vi "From_trubine.vi"(8 "error in (no error)":errorcluster) -> (0 "error out":errorcluster)   [LabVIEW 2022 SP3, in "SI657.lvclass"]
uses:
  SI657.lvclass
  SI656/SI656.lvclass
  SI657.lvclass/SI657.ctl
panel:
  out "Switch Ps-Ps_d":dbl
  out "PG target SP":dbl
  out "PG eff SP":dbl
  out "SI656 out":refnum<class "SI656.lvclass">
  in  "SI656.lvclass":refnum<class "SI656.lvclass">
  in  "Set Params 4":T1
  in  "Set Params 3":T1
  in  "Set Params 2":T1
  in  "Set Params":T1
  out "SI657.lvclass out":refnum<class "SI657.lvclass">
  in  "SI657.lvclass":refnum<class "SI657.lvclass">
  in  "3 MYA01 DU001 XQ10":dbl
  in  "3 MYA01 DU001 XQ11":dbl
  in  "3 MYA01 DU001 XQ13":dbl
  in  "3 MYA01 DU001 XQ12":dbl
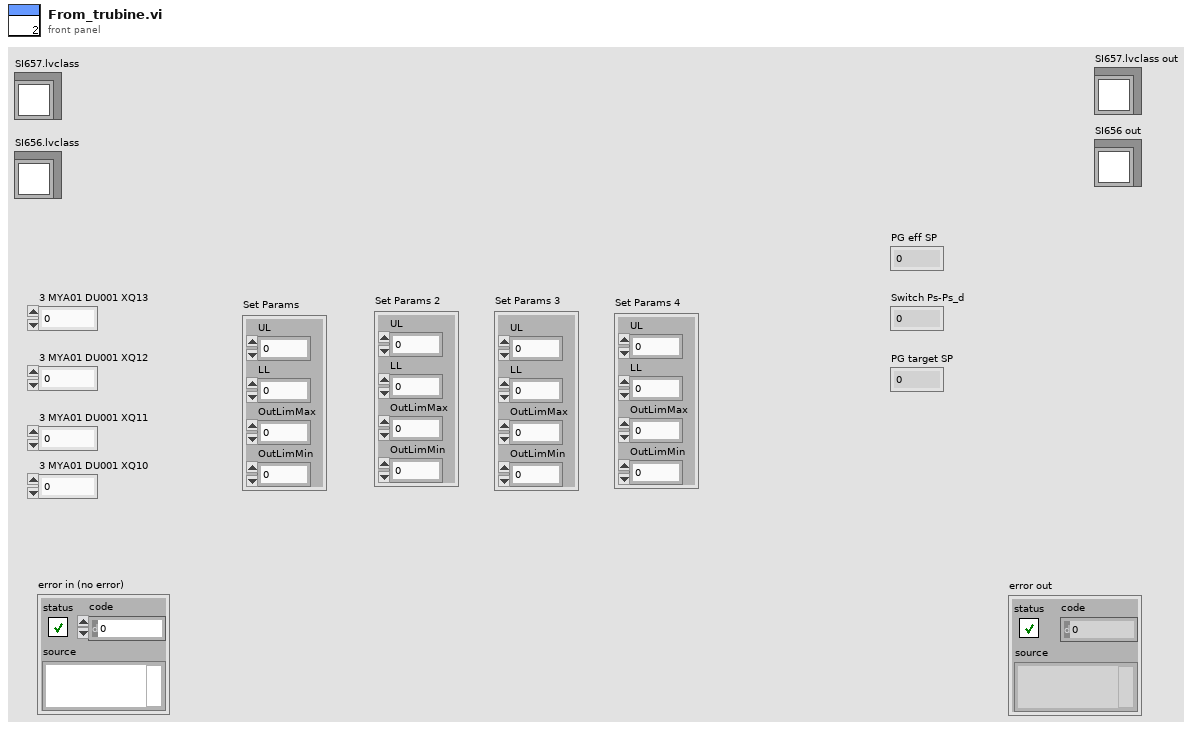
[diagram p1: front panel]
types:
  T1 = cluster{"UL":dbl, "LL":dbl, "OutLimMax":dbl, "OutLimMin":dbl}
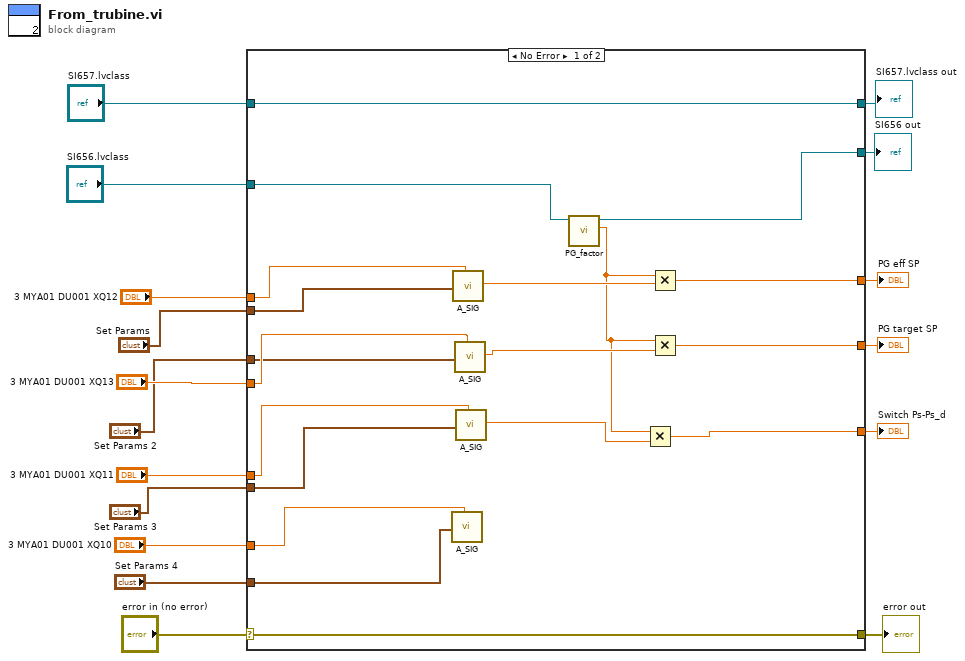
[diagram p0: block diagram]
diagram:
  n1 = case shown="No Error" "error in (no error)" {
    selector: "error in (no error)" -> [w36 w37]
    tunnel: [w36 w37] -> w16
    tunnel: "3 MYA01 DU001 XQ12" -> [w34 _]
    tunnel: "3 MYA01 DU001 XQ13" -> [w33 _]
    tunnel: "3 MYA01 DU001 XQ11" -> [w32 _]
    tunnel: "3 MYA01 DU001 XQ10" -> [w31 _]
    tunnel: "SI657.lvclass" -> [w35 _]
    tunnel: [w35 _] -> w10
    tunnel: "Set Params" -> [w30 _]
    tunnel: "Set Params 2" -> [w29 _]
    tunnel: "Set Params 3" -> [w28 _]
    tunnel: "Set Params 4" -> [w27 _]
    tunnel: "SI656.lvclass" -> [w26 _]
    tunnel: [w25 _] -> w4
    tunnel: [w23 _] -> w3
    tunnel: [w21 _] -> w2
    tunnel: [w18 _] -> w1
    frame No Error {
      n2 = call "A_SIG.vi"("Set Params"=w27, "Input"=w31) -> ()  [unwired: 16 in, 2 out]
      n3 = call "A_SIG.vi"("Set Params"=w30, "Input"=w34) -> ("A_SIG_out"=w24:dbl)  [unwired: 16 in, 1 out]
      n4 = call "A_SIG.vi"("Set Params"=w29, "Input"=w33) -> ("A_SIG_out"=w22:dbl)  [unwired: 16 in, 1 out]
      n5 = call "A_SIG.vi"("Set Params"=w28, "Input"=w32) -> ("A_SIG_out"=w19:dbl)  [unwired: 16 in, 1 out]
      n6 = call "PG_factor.vi"("SI656 in"=w26) -> ("PG Factor"=w20:dbl, "SI656 out"=w25:refnum<class "SI656.lvclass">)  [unwired: 8 in, 1 out]
      n7 = Multiply(x=w20, y=w19) -> (x*y=w18:dbl)
      n8 = Multiply(x=w20, y=w24) -> (x*y=w23:dbl)
      n9 = Multiply(x=w20, y=w22) -> (x*y=w21:dbl)
    }
    frame Error {
    }
  }
  "error out" <- w16
  "SI657.lvclass out" <- w10
  "SI656 out" <- w4
  "PG eff SP" <- w3
  "PG target SP" <- w2
  "Switch Ps-Ps_d" <- w1
